vi "Read Test.vi"() -> ()   [LabVIEW 2019, in "SharedVariableWrapper.lvclass"]
uses:
  SharedVariableWrapper.lvclass
  SharedVariableWrapper.lvclass/SharedVariableWrapper.ctl
  78131cf0-57b9-4322-b737-fe0b31e0abb3.vi
  d8354c83-9461-4e26-96e5-08e4d70f2563.vi
  d8354c83-9461-4e26-96e5-08e4d70f2563.vi/3ecd938c-f3ff-49ee-83ba-9793bc87be91.vi
  Write Var Info.vi
  Read Var Info.vi
  Read connection str.vi
  <userlib>/_OpenG.lib/time/time.llb/Tick Count (ms)__ogtk.vi
panel:
  in  "update timeout":dbl
  out "Updated":bool
  out "Counter":u64
  in  "stop":bool
  out "connected":bool
  out "dt read":u32
  out "error out 2":errorcluster
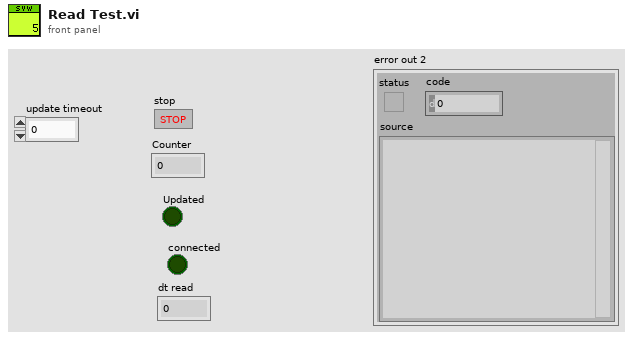
[diagram p1: front panel]
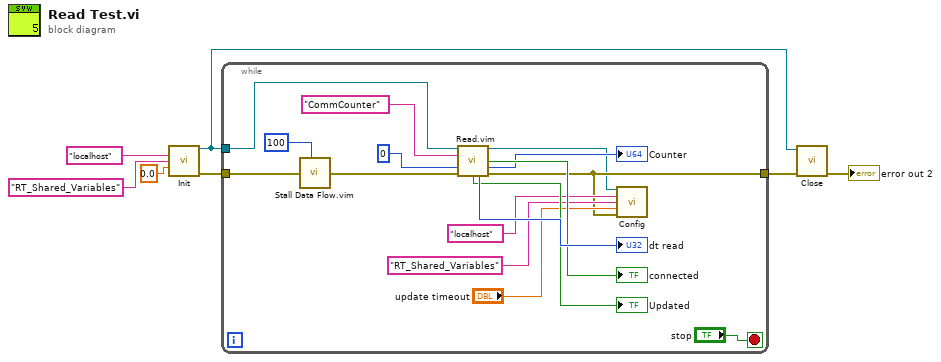
[diagram p0: block diagram]
diagram:
  n1 = call "Init.vi"("host"="localhost", "lib"="RT_Shared_Variables", "update timeout"=0.0) -> ("SVW"=w1:refnum<class "SharedVariableWrapper.lvclass">, "error out"=w3:errorcluster)  [unwired: 11 in]
  n2 = while {
    tunnel: [w13] -> w5
    tunnel: w3 -> [w21]
    tunnel: w1 -> [w9]
    stop <- "stop" stop-if-true
    n3 = call "Stall Data Flow.vim"("value in"=w21, "milliseconds to wait"=u32 100) -> ("value out"=w11:errorcluster)  [unwired: 1 out]
    n4 = call "Read.vim"("SharedVariableWrapper in"=w9, "name"="CommCounter", "DataType"=u64 0, "error in (no error)"=w11) -> ("SharedVariableWrapper out"=w12:refnum<class "SharedVariableWrapper.lvclass">, "connected"=→"connected":bool, "data out"=→"Counter":u64, "Updated"=→"Updated":bool, "dt read"=→"dt read":u32, "error out"=w13:errorcluster)  [unwired: 5 in, 1 out]
    n5 = call "Config.vi"("SharedVariableWrapper in"=w12, "host"="localhost", "lib"="RT_Shared_Variables", "update timeout"="update timeout", "error in"=w13) -> ()  [unwired: 9 in, 2 out]
  }
  n6 = call "Close.vi"("error in (no error)"=w5, "SharedVariableWrapper in"=w1) -> ("error out"=→"error out 2":errorcluster)  [unwired: 8 in, 1 out]
